vi "View Print Save.vi"(8 "error in (no error)":errorcluster, 9 "Plot ID in":T1 format="%x", 10 "appended path":path, 11 "Picture in":refnum<vi>) -> (0 "error out":errorcluster, 3 "Picture":picture)   [LabVIEW 2020]
uses:
  <vilib>/Heliosphere Research LLC/Advanced Plotting Toolkit/typedefs/PlotID.ctl
  <vilib>/Heliosphere Research LLC/Advanced Plotting Toolkit/Advanced Plotting Toolkit.lvlib
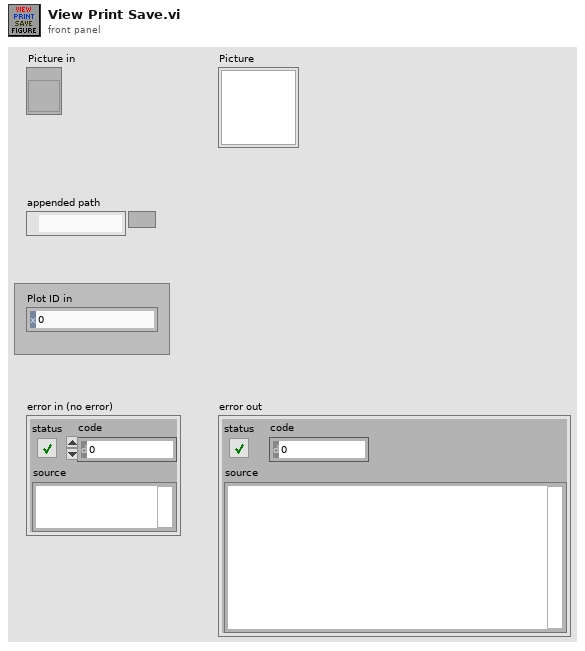
[diagram p1: front panel]
types:
  T1 = typedef "Advanced Plotting Toolkit.lvlib/PlotID.ctl" = i32
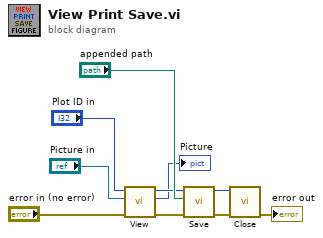
[diagram p0: block diagram]
diagram:
  n1 = call <vilib>:"View.vi"("error in (no error)"="error in (no error)", "Ref for Sizing"="Picture in", "Plot ID"="Plot ID in") -> ("error out"=w4:errorcluster, "Picture"=→"Picture":picture, "Plot ID Out"=w7:T1)  [unwired: 6 in]
  n2 = call <vilib>:"Save.vi"("error in (no error)"=w4, "Path"="appended path", "Plot ID In"=w7) -> ("error out"=w5:errorcluster, "Plot ID Out"=w6:T1)  [unwired: 7 in]
  n3 = call <vilib>:"Close.vi"("error in (no error)"=w5, "Plot ID"=w6) -> ("error out"=→"error out":errorcluster)  [unwired: 9 in]
